vi "Configure Trigger Scope.vi"(8 "error in (no error)":errorcluster, 10 "Scope (0: All Channels)":i32(ring) items=["All Channels", "Active Channel"], 11 "VISA resource name":refnum<visa-resource-name>) -> (0 "error out":errorcluster, 3 "VISA resource name out":refnum<visa-resource-name>)   [LabVIEW 2020, in "Agilent ENA Series.lvlib"]
doc: "Configures trigger scope."
uses:
  <instrlib>/Agilent ENA Series/Agilent ENA Series.lvlib
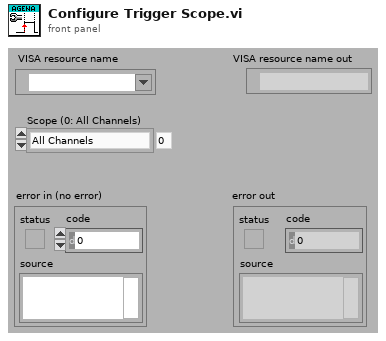
[diagram p1: front panel]
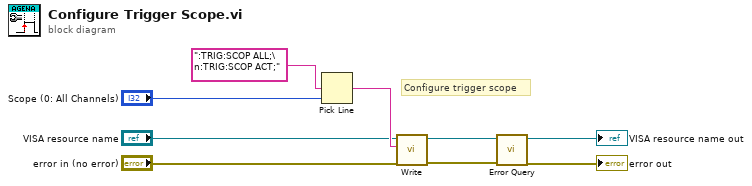
[diagram p0: block diagram]
diagram:
  # "Configure trigger scope"
  n1 = Pick Line(multi-line string=":TRIG:SCOP ALL;\n:TRIG:SCOP ACT;", line index="Scope (0: All Channels)") -> (output string=w5:string)  [unwired: 1 out]
  n2 = call <instrlib>:"Write.vi"("error in (no error)"="error in (no error)", "String ()"=w5, "VISA resource name"="VISA resource name") -> ("error out"=w1:errorcluster, "VISA resource name out"=w2:refnum<visa-resource-name>)  [unwired: 6 in, 1 out]
  n3 = call <instrlib>:"Error Query.vi"("error in (no error)"=w1, "VISA resource name"=w2) -> ("error out"=→"error out":errorcluster, "VISA resource name out"=→"VISA resource name out":refnum<visa-resource-name>)  [unwired: 8 out]
